vi "Write ch_units.vi"(8 "error in (no error)":errorcluster, 10 "ch_units":string[](array[string]), 11 "Sim DiscreteIO in":refnum<class "Sim DiscreteIO.lvclass">) -> (0 "error out":errorcluster, 3 "Sim DiscreteIO out":refnum<class "Sim DiscreteIO.lvclass">)   [LabVIEW 2021, in "Sim DiscreteIO.lvclass"]
uses:
  Sim DiscreteIO.lvclass
  Sim DiscreteIO.lvclass/Sim DiscreteIO.ctl
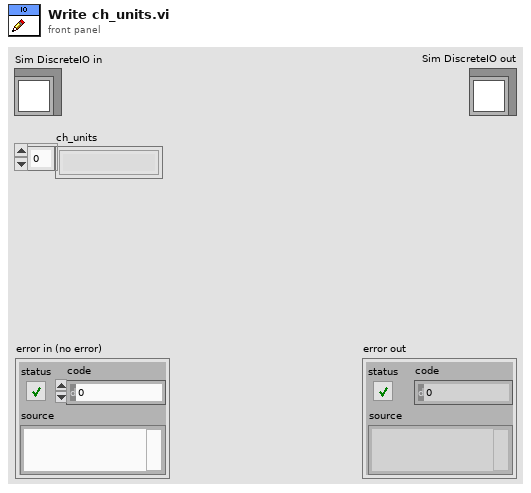
[diagram p1: front panel]
types:
  T1 = typedef "Sim DiscreteIO.lvclass/DVR.ctl" = cluster{"ch_labels":string[], "_PARMS":T2, "Initialized?":bool, "occurrence":refnum<k4>}
  T2 = typedef "Sim DiscreteIO.lvclass/_PARMS.ctl" = cluster{"ch_units":string[], "ch_alias":string[]}
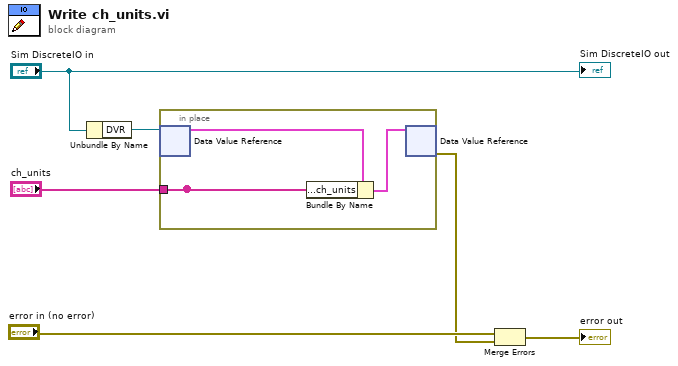
[diagram p0: block diagram]
diagram:
  n1 = Unbundle By Name ("DVR Unbundle")("Sim DiscreteIO in") -> ("DVR"=w2:refnum<data-value>)
  n2 = in-place "In Place Element Structure" {
    in-place-border: [w7] -> _
    in-place-border: "ch_units" -> [w7]
    n3 = in-place-dvr #1(w2) -> (w9:T1)  [unwired: 1 out]
    n4 = Bundle By Name ("Item Bundle")(cluster=w9, "_PARMS.ch_units"=w7) -> (w8:T1)
    n5 = in-place-dvr #1(w8) -> (w3:errorcluster)  [unwired: 1 out]
  }
  n6 = Merge Errors("error in (no error)", w3) -> (→"error out":errorcluster)
  "Sim DiscreteIO out" <- "Sim DiscreteIO in"
